vi "Page_Version_Initialize.vi"(6 "output cluster":T1, 8 "error in (no error)":errorcluster, 11 "AB_DepPackedLibrary in":refnum<class "AB_DepPackedLibrary.lvclass">) -> (0 "error out":errorcluster, 3 "AB_DepPackedLibrary out":refnum<class "AB_DepPackedLibrary.lvclass">)   [LabVIEW 2020, in "AB_DepPackedLibrary.lvclass"]
uses:
  <vilib>/AppBuilder/AB_Classes/DepPackedLib/AB_DepPackedLibrary.lvclass
  e:/builds/penguin/labview/branches/2020/dev/dist/vi.lib/AppBuilder/AB_Classes/Build/AB_Build.lvclass
  <resource>/Framework/Providers/Builds/AppBuilder/AB_UI_Page_Version_References.ctl
  <vilib>/AppBuilder/AB_Classes/Deployment/AB_Deployment.lvlib
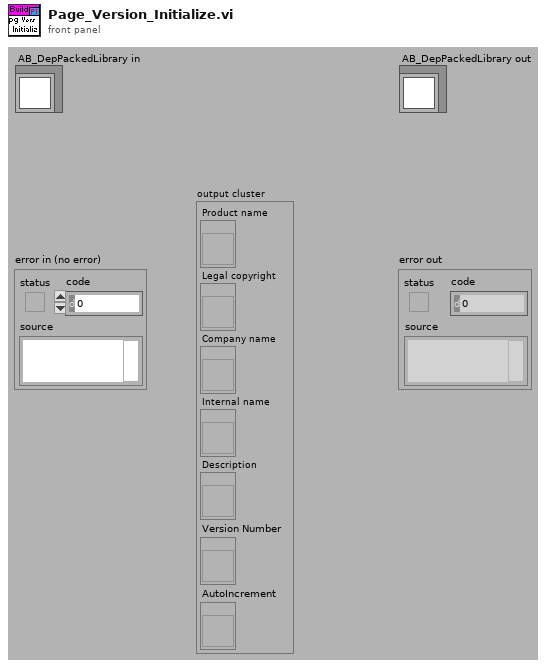
[diagram p1: front panel]
types:
  T1 = typedef "AB_UI_Page_Version_References.ctl" = cluster{"Product name":refnum<vi>, "Legal copyright":refnum<vi>, "Company name":refnum<vi>, "Internal name":refnum<vi>, "Description":refnum<vi>, "Version Number":refnum<vi>, "AutoIncrement":refnum<vi>}
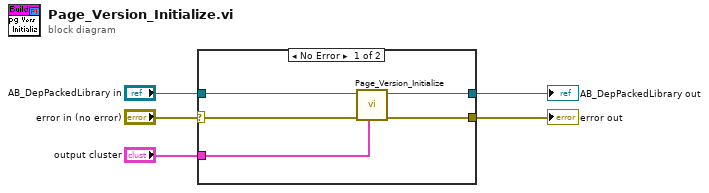
[diagram p0: block diagram]
diagram:
  n1 = case shown="No Error" "error in (no error)" {
    selector: "error in (no error)" -> [w8 w11]
    tunnel: "AB_DepPackedLibrary in" -> [w10 w12]
    tunnel: [w9 w12] -> w4
    tunnel: [w7 w11] -> w3
    tunnel: "output cluster" -> [w6 _]
    frame No Error {
      n2 = call <vilib>:"Page_Version_Initialize.vi"("output cluster"=w6, "error in (no error)"=w8, "Build in"=w10) -> ("error out"=w7:errorcluster, "Build out"=w9:refnum<class "AB_DepPackedLibrary.lvclass">)  [unwired: 7 in]
    }
    frame Error {
    }
  }
  "error out" <- w3
  "AB_DepPackedLibrary out" <- w4
